vi "EncoderRightDrive.vi"(6 "Zero":bool, 7 "Update":bool, 11 "Position_in":i32) -> (3 "Position_out":i32)   [LabVIEW 2015]
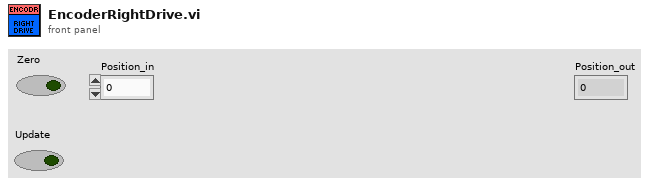
[diagram p1: front panel]
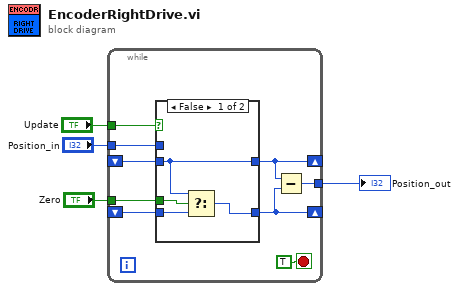
[diagram p0: block diagram]
diagram:
  n1 = while {
    shift-right: [w7] -> _
    shift-left: _ -> [w13]
    tunnel: "Position_in" -> [w12]
    tunnel: "Update" -> [w11]
    shift-right: [w6] -> _
    shift-left: _ -> [w8]
    tunnel: "Zero" -> [w9]
    tunnel: [w5] -> w1
    stop <- TRUE stop-if-true
    n2 = case shown="False" w11 {
      tunnel: w13 -> [w15 _]
      tunnel: [w15 w19] -> w7
      tunnel: w12 -> [_ w19]
      tunnel: w9 -> [w17 _]
      tunnel: w8 -> [w16 w18]
      tunnel: [w14 w18] -> w6
      frame False {
        n3 = Select(t=w15, s=w17, f=w16) -> (s? t:f=w14:i32)
      }
      frame True {
      }
    }
    n4 = Subtract(x=w7, y=w6) -> (x-y=w5:i32)
  }
  "Position_out" <- w1
